vi "Set Stop Trigger (Formula).vi"(7 "Post-Trigger Duration (0 s)":dbl, 8 "error in (no error)":errorcluster, 9 "Variable Mappings":T2[](array[typedef]), 10 "Trigger Condition":string, 11 "Data Logging Specification Ref in":T1) -> (0 "error out":errorcluster, 3 "Data Logging Specification Ref out":T1)   [LabVIEW 2020, in "NI_VS Data Logging API.lvlib"]
doc: "Specifies a stop trigger condition that occurs when the formula specified in the <b>Trigger Condition</b> input evaluates to true. This formula must be a Boolean expression. The variables used in the expression must be valid identifiers. Use the <b>Variable Mappings</b> input to map the variables used in the expression to system definition channels, whose values will be used to evaluate the expression.\n\nUse the <b>Post-Trigger Duration</b> input to specify the post-trigger duration, which indicates the duration in seconds of data that is logged after the stop trigger condition occurs."
uses:
  <vilib>/NI VeriStand/Execution/DataLogging/NI_VS Data Logging API.lvlib
  <vilib>/NI VeriStand/Execution/DataLogging/DataLoggingSpecification Ref.ctl
  NationalInstruments.VeriStand.ClientAPI
  <vilib>/NI VeriStand/Execution/DataLogging/Variable Mapping.ctl
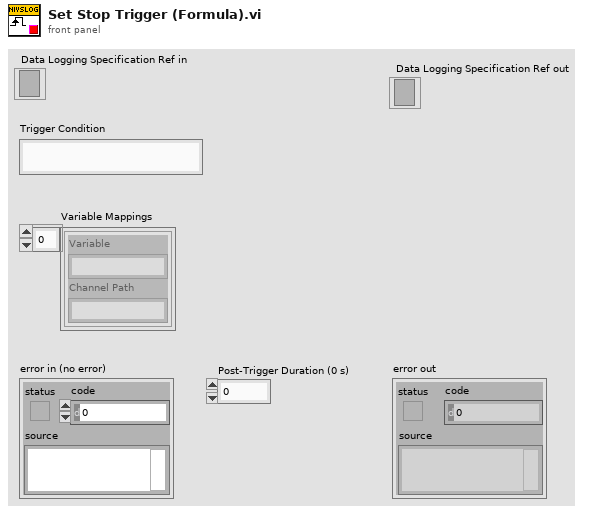
[diagram p1: front panel]
types:
  T1 = typedef "NI_VS Data Logging API.lvlib/DataLoggingSpecification Ref.ctl" = refnum<k24>
  T2 = typedef "NI_VS Data Logging API.lvlib/Variable Mapping.ctl" = cluster{"Variable":string, "Channel Path":string}
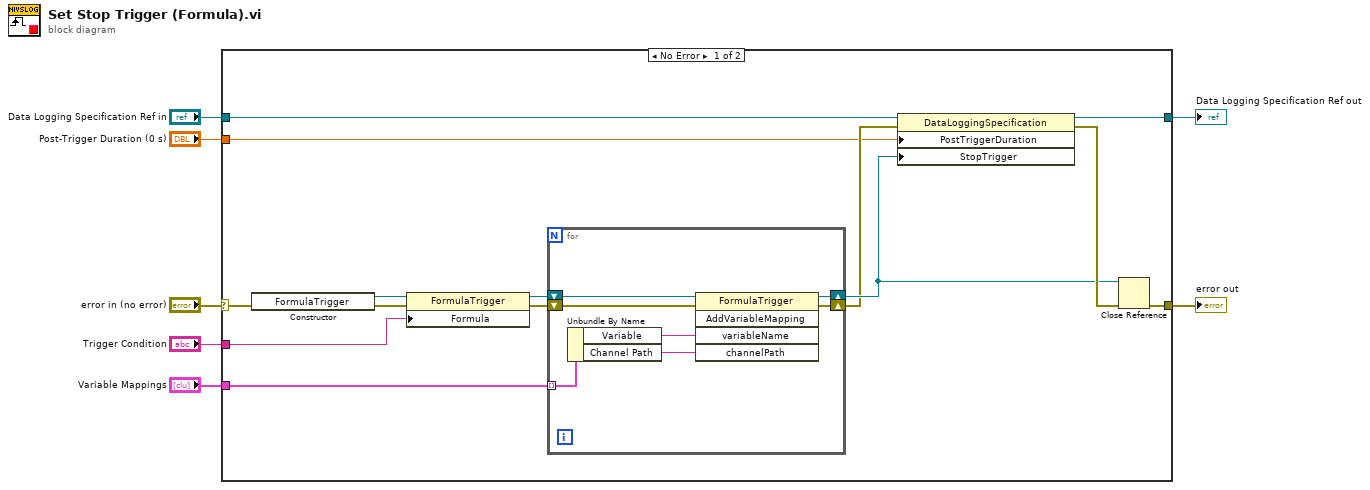
[diagram p0: block diagram]
diagram:
  n1 = case shown="No Error" "error in (no error)" {
    selector: "error in (no error)" -> [w15 w30]
    tunnel: "Variable Mappings" -> [w14 _]
    tunnel: "Trigger Condition" -> [w13 _]
    tunnel: "Data Logging Specification Ref in" -> [w20 w29]
    tunnel: [w10 w29] -> w4
    tunnel: [w9 w30] -> w3
    tunnel: "Post-Trigger Duration (0 s)" -> [w8 _]
    frame No Error {
      n2 = constructor class="FormulaTrigger"(error in=w15) -> (reference out=w19:refnum<k24>, error out=w18:errorcluster)  [unwired: 2 in, 1 out]
      n3 = property class="FormulaTrigger"(reference=w19, error in=w18, "Formula"=w13) -> (reference out=w17:refnum<k24>, error out=w16:errorcluster)
      n4 = for {
        shift-right: [w26] -> w12
        shift-left: w17 -> [w28]
        shift-right: [w25] -> w11
        shift-left: w16 -> [w27]
        tunnel: w14 -> [w24] mode=indexing
        n5 = Unbundle By Name(w24) -> ("Variable"=w23:string, "Channel Path"=w22:string)
        n6 = invoke class="FormulaTrigger" method="AddVariableMapping"(reference=w28, error in=w27, "variableName"=w23, "channelPath"=w22) -> (reference out=w26:refnum<k24>, error out=w25:errorcluster)  [unwired: 1 in, 3 out]
      }
      n7 = property class="DataLoggingSpecification"(reference=w20, error in=w11, "PostTriggerDuration"=w8, "StopTrigger"=w12) -> (reference out=w10:T1, error out=w21:errorcluster)
      n8 = Close Reference(reference=w12, error in (no error)=w21) -> (error out=w9:errorcluster)
    }
    frame Error {
    }
  }
  "error out" <- w3
  "Data Logging Specification Ref out" <- w4
